vi "CheckSubmittedBooks.vi"(6 "Username":string, 7 "Remote Path":string="dropBox/", 8 "Books":refnum<vi>) -> (0 "error out":errorcluster, 1 "graded":string, 2 "submitted":string[][](array[string]), 4 "dropBox":string, 5 "symbols":i16[](array[numeric]))   [LabVIEW 2012]
panel:
  in  "Tab Control":enum32{"dropBox", "gradedAssignment"}(tab)
  out "graded":string[][](array[string])
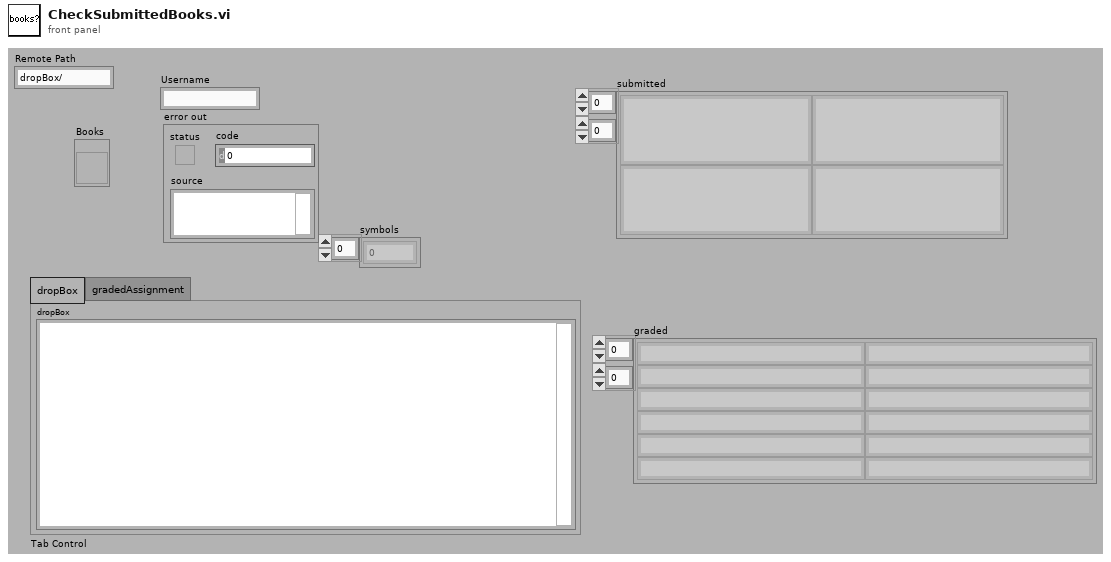
[diagram p1: front panel]
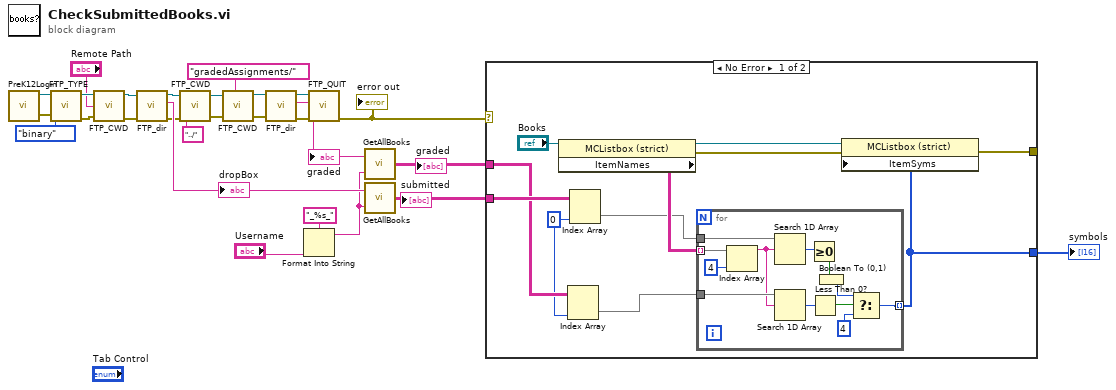
[diagram p0: block diagram]
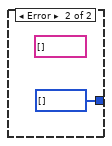
[diagram p2: hidden frame]
diagram:
  n1 = call <userlib>:"PreK12Login.vi"() -> ("error out"=w25:errorcluster, "connection ID out"=w26:refnum<k5>)  [unwired: 2 in]
  n2 = call <userlib>:"FTP_TYPE.vi"("connection ID"=w26, "type (query)"=enum16{"(query)", "ASCII", "binary"}."binary", "error in"=w25) -> ("connection ID out"=w24:refnum<k5>, "error out"=w23:errorcluster)  [unwired: 2 out]
  n3 = call <userlib>:"FTP_CWD.vi"("connection ID"=w24, "path"="Remote Path", "error in"=w23) -> ("connection ID out"=w22:refnum<k5>, "error out"=w21:errorcluster)  [unwired: 2 out]
  n4 = call <userlib>:"FTP_dir.vi"("connection ID"=w22, "error in"=w21) -> ("connection ID out"=w14:refnum<k5>, "reply string"=w18:string, "error out"=w13:errorcluster)  [unwired: 2 out]
  "dropBox" <- w18
  n5 = call <userlib>:"FTP_CWD.vi"("connection ID"=w14, "path"="../" ("Remote Path"), "error in"=w13) -> ("connection ID out"=w7:refnum<k5>, "error out"=w2:errorcluster)  [unwired: 2 out]
  n6 = call <userlib>:"FTP_CWD.vi"("connection ID"=w7, "path"="gradedAssignments/", "error in"=w2) -> ("connection ID out"=w4:refnum<k5>, "error out"=w3:errorcluster)  [unwired: 2 out]
  n7 = call <userlib>:"FTP_dir.vi"("connection ID"=w4, "error in"=w3) -> ("connection ID out"=w11:refnum<k5>, "reply string"=w1:string, "error out"=w10:errorcluster)  [unwired: 2 out]
  "graded" <- w1
  n8 = Format Into String(format string="_%s_", "Username") -> (resulting string=w9:string)  [unwired: 2 in, 1 out]
  n9 = call <userlib>:"FTP_QUIT.vi"("connection ID"=w11, "error in"=w10) -> ("error out"=w16:errorcluster)  [unwired: 3 out]
  "error out" <- w16
  n10 = call <userlib>:"GetAllBooks.vi"("Author"=w9, "directory"=w1) -> ("books"=w5:string[][])
  "graded" <- w5
  n11 = call <userlib>:"GetAllBooks.vi"("Author"=w9, "directory"=w18) -> ("books"=w6:string[][])
  "submitted" <- w6
  n12 = case shown="No Error" w16 {
    tunnel: w6 -> [w37 _]
    tunnel: [w31 i16[] []] -> w15
    tunnel: [w33 _] -> _
    tunnel: w5 -> [w32 _]
    frame No Error {
      w28 = 0 ("disabled index (col)")
      n13 = property class="MCListbox (strict)"(reference="Books") -> (reference out=w35:refnum<vi>, error out=w34:errorcluster, "ItemNames"=w36:string[][])  [unwired: 1 in]
      n14 = Index Array(array=w32, index (col)=w28) -> (element=w29:string[])  [unwired: 1 in]
      n15 = Index Array(array=w37, index (col)=w28) -> (element=w30:string[])  [unwired: 1 in]
      n16 = for {
        tunnel: w30 -> [w50]
        tunnel: w36 -> [w49] mode=indexing
        tunnel: w29 -> [w47]
        tunnel: [w42] -> w31 mode=indexing
        n17 = Index Array(array=w49, index=4) -> (element=w46:string)
        n18 = Search 1D Array(1D array=w50, element=w46) -> (index of element=w48:i32)  [unwired: 1 out]
        n19 = Search 1D Array(1D array=w47, element=w46) -> (index of element=w45:i32)  [unwired: 1 out]
        n20 = Greater Or Equal To 0?(x=w48) -> (x >= 0?=w43:bool)
        n21 = Less Than 0?(x=w45) -> (x < 0?=w44:bool)
        n22 = Boolean To (0,1)(Boolean=w43) -> (0, 1=w41:i16)
        n23 = Select(t=w41, s=w44, f=4) -> (s? t:f=w42:i32)
      }
      n24 = property class="MCListbox (strict)"(reference=w35, error in=w34, "ItemSyms"=w31) -> (error out=w33:errorcluster)  [unwired: 1 out]
    }
    frame Error {
      (unwired) string[] [] ("Array")
    }
  }
  "symbols" <- w15
